vi "Check Prompt Q.vi"(8 "error in (no error)":errorcluster, 11 "LoggingControl in":refnum<class "GroupLoggingControl.lvclass">) -> (0 "error out":errorcluster, 3 "LoggingControl out":refnum<class "GroupLoggingControl.lvclass">)   [LabVIEW 2020, in "VolatusGUIElements.lvlib" / "GroupLoggingControl.lvclass"]
uses:
  GroupLoggingControl.lvclass
  GroupLoggingControl.lvclass/GroupLoggingControl.ctl
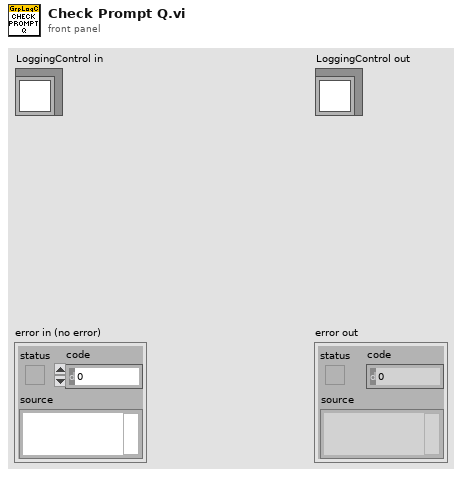
[diagram p1: front panel]
types:
  T1 = typedef "VolatusGUIElements.lvlib/GroupLoggingControl.lvclass/Prompt Result.ctl" = cluster{"Action":T2, "Series":string, "Timestamp":string}
  T2 = typedef "VolatusGUIElements.lvlib/GroupLoggingControl.lvclass/Prompt Action.ctl" = enum16{"Cancelled", "Started"}
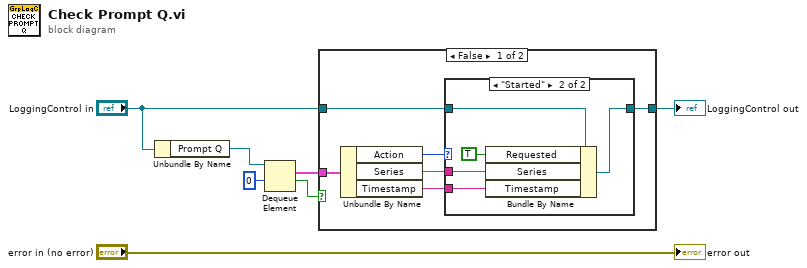
[diagram p0: block diagram]
diagram:
  n1 = Unbundle By Name("LoggingControl in") -> ("Prompt Q"=w6:refnum<queue>)
  n2 = Dequeue Element(queue=w6, timeout in ms (-1)=0) -> (element=w2:T1, timed out?=w3:bool)  [unwired: 1 in, 2 out]
  n3 = case shown="False" w3 {
    tunnel: "LoggingControl in" -> [w12 w20]
    tunnel: w2 -> [w13 _]
    tunnel: [w8 w20] -> w1
    frame False {
      n4 = Unbundle By Name(w13) -> ("Action"=w11:T2, "Series"=w10:string, "Timestamp"=w9:string)
      n5 = case shown="\"Started\"" w11 {
        tunnel: w12 -> [w14 w19]
        tunnel: w10 -> [_ w18]
        tunnel: w9 -> [_ w16]
        tunnel: [w14 w15] -> w8
        frame "Cancelled" {
        }
        frame "Started" {
          n6 = Bundle By Name(cluster=w19, "Requested"=TRUE ("State.Requested"), "Series"=w18, "Timestamp"=w16) -> (w15:refnum<class "GroupLoggingControl.lvclass">)
        }
      }
    }
    frame True {
    }
  }
  "LoggingControl out" <- w1
  "error out" <- "error in (no error)"
